vi "Get Bar Color.vi"(4 "Y Dimension":i32, 6 "X Dimension":i32, 7 "Opacity":sgl, 9 "Draw Mode":T2(ring)=enum."Quads", 11 "Color Pair Array":cluster{"Color":u32, "String":string}[](array[cluster])) -> (1 "Color Binding Mode":T1(ring)=enum."Per Primitive", 3 "Color Array":cluster{"R":sgl, "G":sgl, "B":sgl, "A":sgl}[](array[cluster]))   [LabVIEW 2020, in "3D Bar.lvclass"]
uses:
  <vilib>/Math Plots/3D Math Plots/3D Bar/3D Bar/3D Bar.lvclass
  <vilib>/picture/3D Picture Control/NI_3D Picture Control.lvlib
  <vilib>/Math Plots/3D Math Plots/3D Plot/3D Plot/3D Plot.lvclass
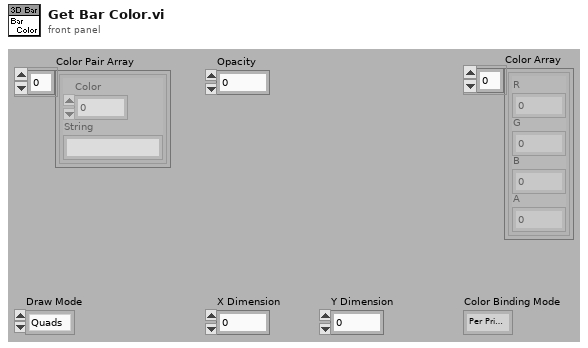
[diagram p1: front panel]
types:
  T1 = enum16{"Overall", "Per Primitive", "Per Vertex", "Binding Off"}
  T2 = enum16{"Points", "Lines", "Line Strip", "Line Loop", "Triangles", "Triangle Strip", "Triangle Fan", "Quads", "Quad Strip", "Polygon"}
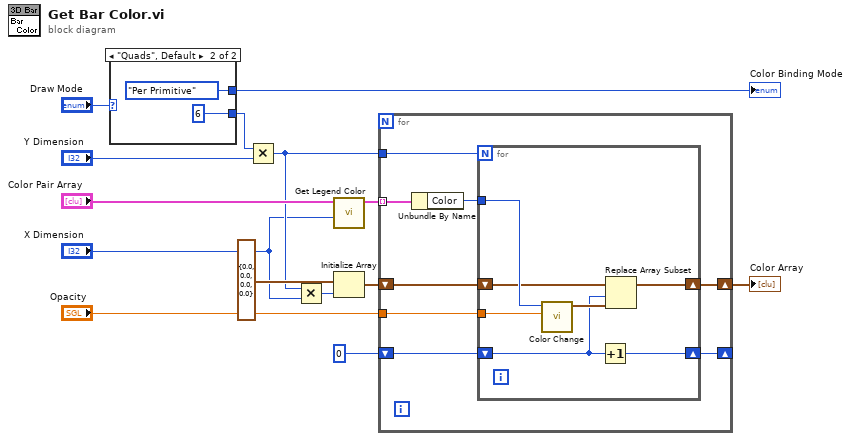
[diagram p0: block diagram]
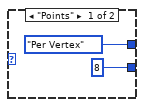
[diagram p2: hidden frame]
diagram:
  n1 = case shown="\"Quads\", Default" "Draw Mode" {
    tunnel: [8 ("y") 6 ("y")] -> w9
    tunnel: [T1."Per Vertex" ("Color Binding Mode") T1."Per Primitive" ("Color Binding Mode")] -> w1
    frame "Points" {
    }
    frame "Quads", Default {
    }
  }
  "Color Binding Mode" <- w1
  n2 = Multiply(x=w9, y="Y Dimension") -> (x*y=w5:i32)
  n3 = Multiply(x=w5, y="X Dimension") -> (x*y=w3:i32)
  n4 = call <vilib>:"Get Legend Color.vi"("Pair Array Length"="X Dimension", "Color Pair Array In"="Color Pair Array") -> ("Color Pair Array Out"=w11:cluster{"Color":u32, "String":string}[])  [unwired: 9 out]
  n5 = Initialize Array(cluster{"R":sgl, "G":sgl, "B":sgl, "A":sgl} {"R"=0.0, "G"=0.0, "B"=0.0, "A"=0.0} ("RGBA"), w3) -> (w6:cluster{"R":sgl, "G":sgl, "B":sgl, "A":sgl}[])
  n6 = for {
    tunnel: "Opacity" -> [w26]
    tunnel: w11 -> [w24] mode=indexing
    tunnel: w5 -> [w22]
    shift-right: [w25] -> w13
    shift-left: w6 -> [w21]
    shift-right: [w20] -> _
    shift-left: 0 ("y") -> [w19]
    n7 = Unbundle By Name(w24) -> ("Color"=w23:u32)
    n8 = for {
      N: w22 -> [_]
      tunnel: w26 -> [w33]
      tunnel: w23 -> [w32]
      shift-right: [w30] -> w25
      shift-left: w21 -> [w31]
      shift-right: [w28] -> w20
      shift-left: w19 -> [w27]
      n9 = call <vilib>:"Color Change.vi"("Alpha"=w33, "Color"=w32) -> ("RGBA"=w29:cluster{"R":sgl, "G":sgl, "B":sgl, "A":sgl})  [unwired: 9 out]
      n10 = Increment(x=w27) -> (x+1=w28:i32)
      n11 = Replace Array Subset(array=w31, new element=w29, index=w27) -> (w30:cluster{"R":sgl, "G":sgl, "B":sgl, "A":sgl}[])
    }
  }
  "Color Array" <- w13
